vi "Read Element of Cubes.vi"(8 "error in (no error)":errorcluster, 10 "index":i32, 11 "Cubes in":refnum<class "Cubes.lvclass">) -> (0 "error out":errorcluster, 2 "Cube":refnum<class "Cube.lvclass">, 3 "Cubes out":refnum<class "Cubes.lvclass">)   [LabVIEW 2019, in "22.lvlib" / "Cubes.lvclass"]
uses:
  Cubes.lvclass
  Cube/Cube.lvclass
  Cubes.lvclass/Cubes.ctl
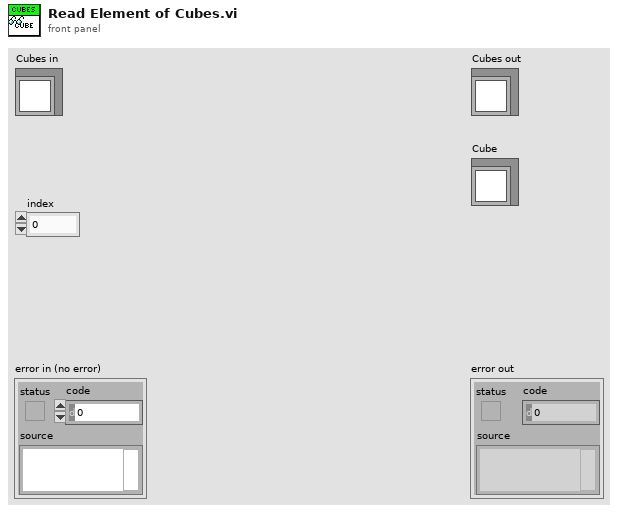
[diagram p1: front panel]
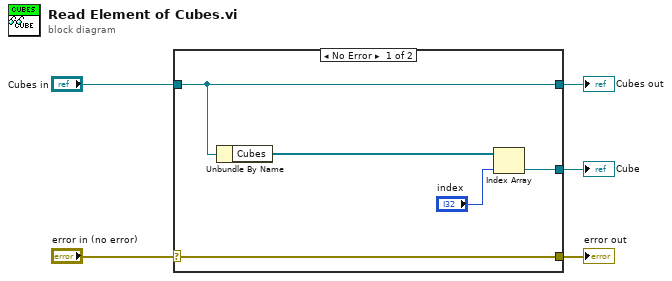
[diagram p0: block diagram]
diagram:
  n1 = case shown="No Error" "error in (no error)" {
    selector: "error in (no error)" -> [w10 w11]
    tunnel: [w10 w11] -> w4
    tunnel: [w9 w12] -> w2
    tunnel: "Cubes in" -> [w9 w12]
    tunnel: [w6 _] -> w1
    frame No Error {
      n2 = Unbundle By Name(w9) -> ("Cubes"=w8:refnum<class "Cube.lvclass">[])
      n3 = Index Array(array=w8, index="index") -> (element=w6:refnum<class "Cube.lvclass">)
    }
    frame Error {
    }
  }
  "error out" <- w4
  "Cubes out" <- w2
  "Cube" <- w1
